vi "inout_map.vi"(9 "Input Sequence":dbl[](array[numeric])) -> (0 "array":string[](array[string]))   [LabVIEW 2021, in "CALIBRATION.lvlib"]
uses:
  CALIBRATION.lvlib
panel:
  out "spreadsheet string":string
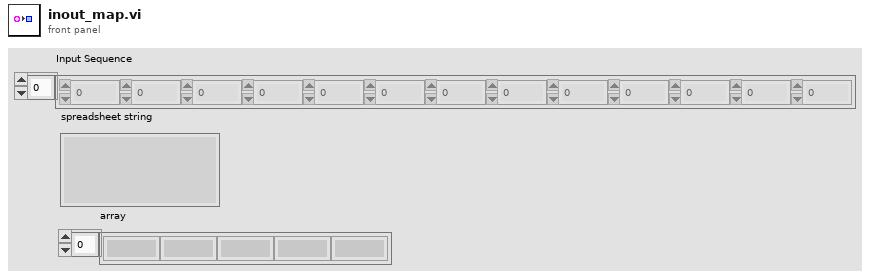
[diagram p1: front panel]
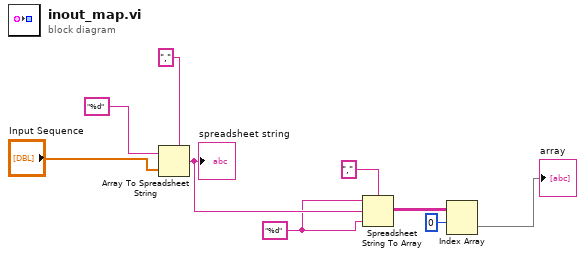
[diagram p0: block diagram]
diagram:
  w4 = "%d" ("format string")
  n1 = Array To Spreadsheet String(delimiter (Tab)=",", array="Input Sequence", 3:"%d" ("format string")) -> (spreadsheet string=w6:string)
  "spreadsheet string" <- w6
  n2 = Spreadsheet String To Array(delimiter (Tab)=",", format string=w4, spreadsheet string=w6, array type (2D Dbl)=w4) -> (array=w3:string[][])
  n3 = Index Array(array=w3, index (row)=0) -> (element=→"array":string[])  [unwired: 1 in]
